vi "V2 Upgrade Refactor Data.vi"() -> (0 "refactor data":T1)   [LabVIEW 2021, in "MeasurementService Editor.lvlib"]
uses:
  MeasurementService Editor.lvlib
  Rename Refactor Mapping Info.ctl
  Rename Refactor Data.ctl
  Rename String Mapping.ctl
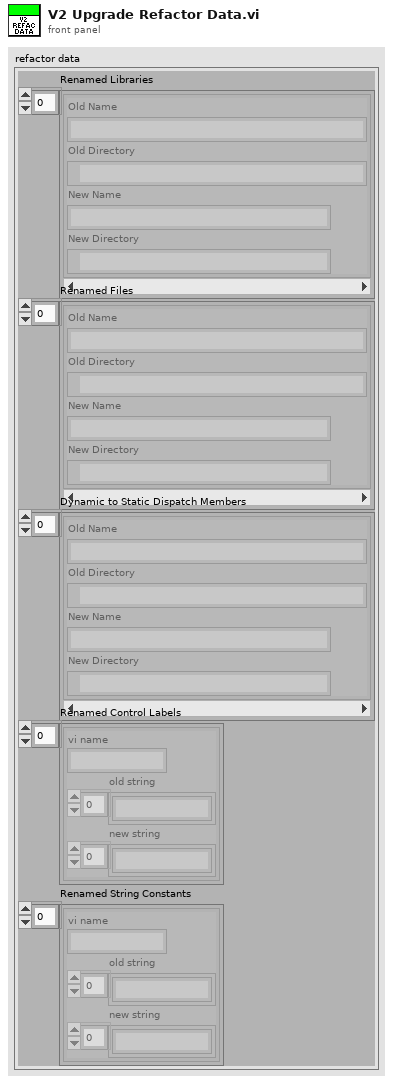
[diagram p1: front panel]
types:
  T1 = typedef "MeasurementService Editor.lvlib/Rename Refactor Data.ctl" = cluster{"Renamed Libraries":T2[], "Renamed Files":T2[], "Dynamic to Static Dispatch Members":T2[], "Renamed Control Labels":T3[], "Renamed String Constants":T3[]}
  T2 = typedef "MeasurementService Editor.lvlib/Rename Refactor Mapping Info.ctl" = cluster{"Old Name":string, "Old Directory":path, "New Name":string, "New Directory":path}
  T3 = typedef "MeasurementService Editor.lvlib/Rename String Mapping.ctl" = cluster{"vi name":string, "old string":string[], "new string":string[]}
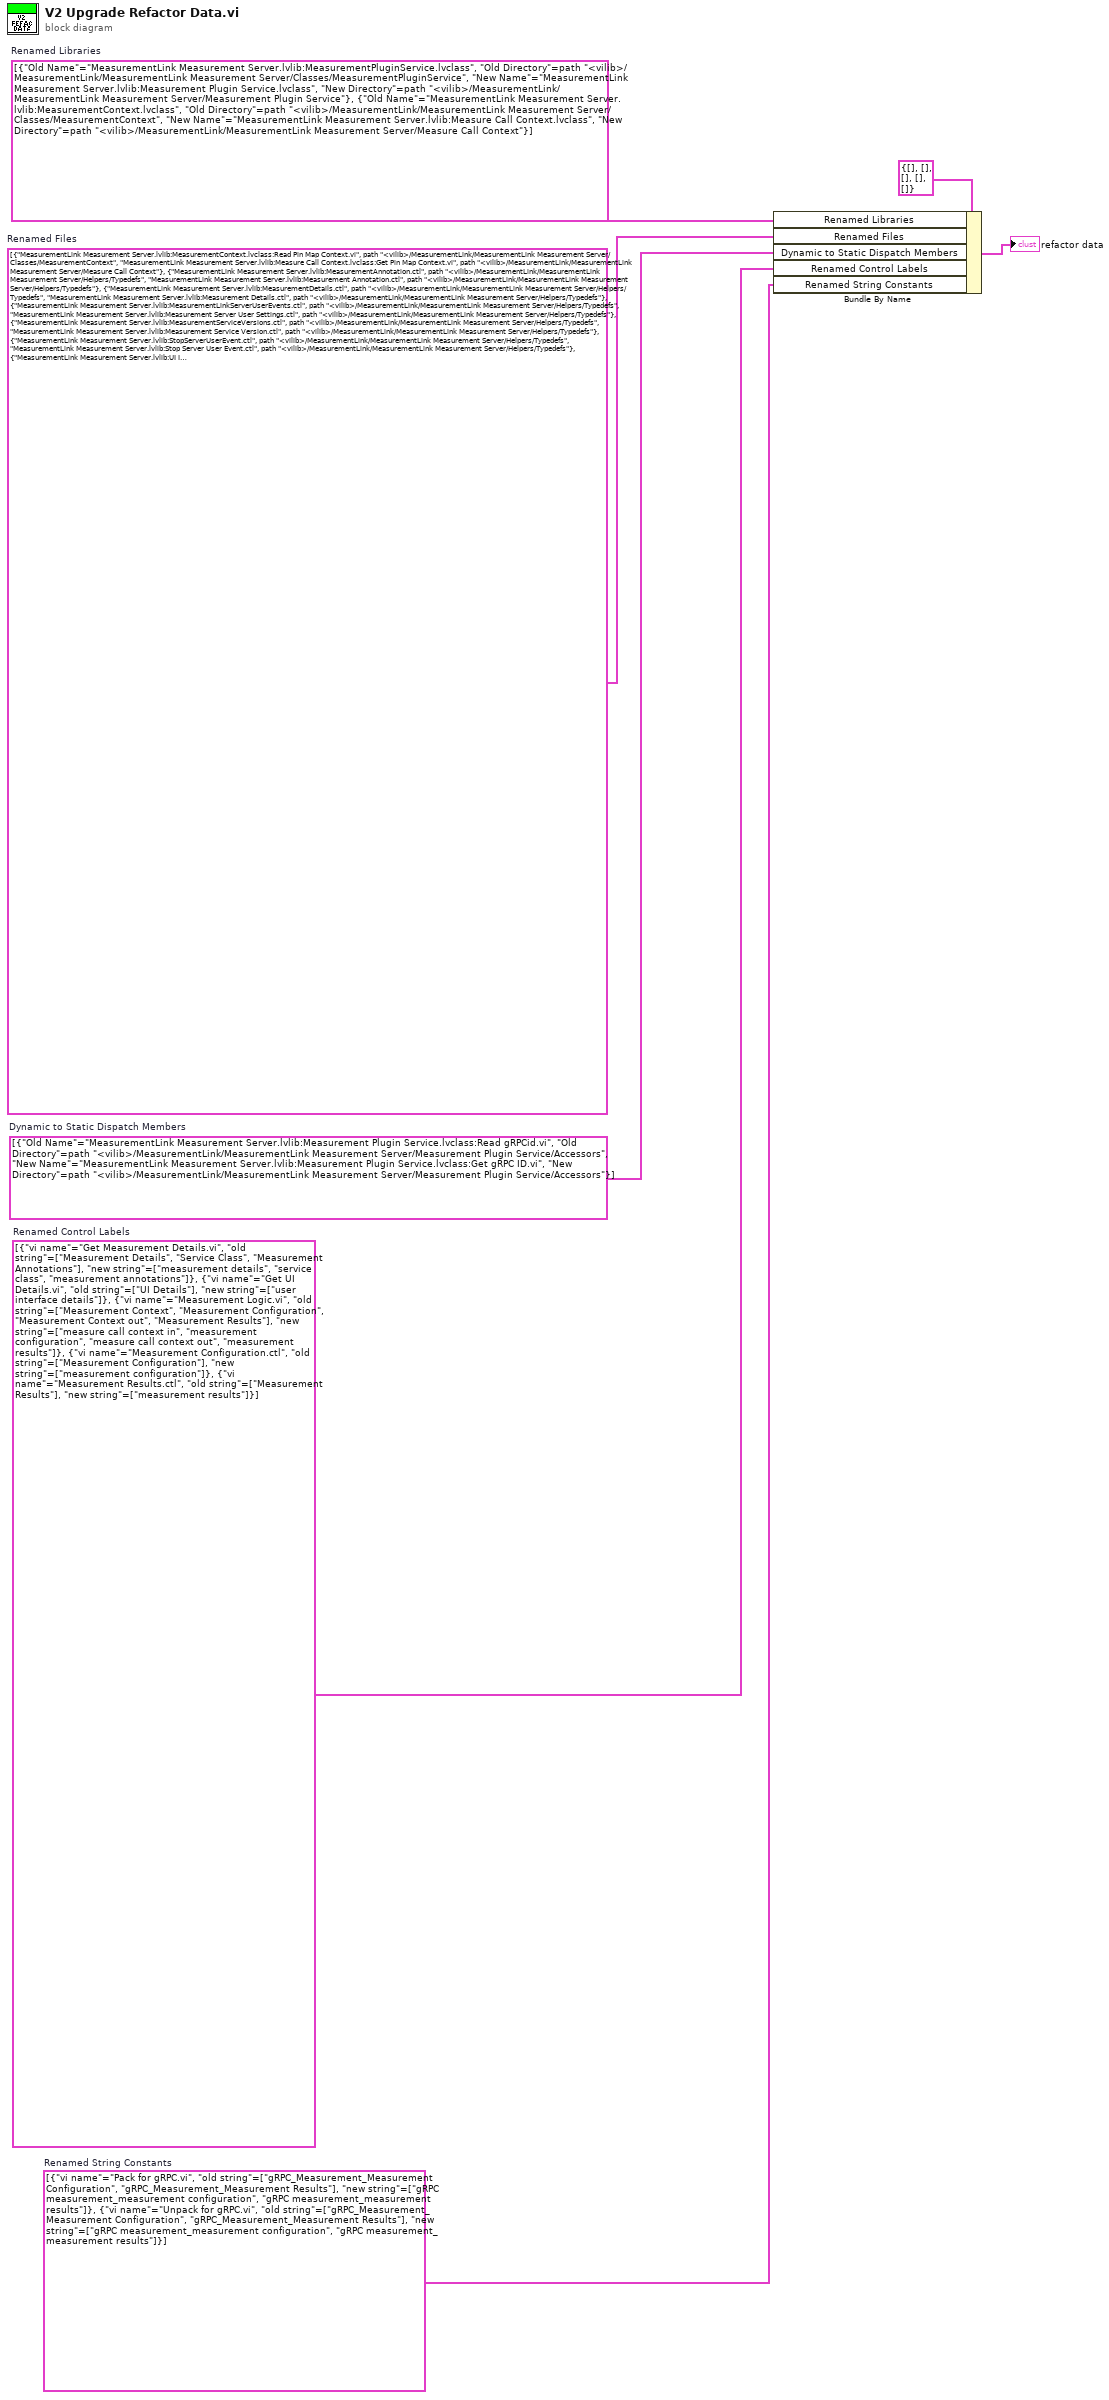
[diagram p0: block diagram]
diagram:
  w1 = T3[] [{"vi name"="Pack for gRPC.vi", "old string"=["gRPC_Measurement_Measurement Configuration", "gRPC_Measurement_Measurement Results"], "new string"=["gRPC measurement_measurement configuration", "gRPC measurement_measurement results"]}, {"vi name"="Unpack for gRPC.vi", "old string"=["gRPC_Measurement_Measurement Configuration", "gRPC_Measurement_Measurement Results"], "new string"=["gRPC measurement_measurement configuration", "gRPC measurement_measurement results"]}]  # Renamed String Constants
  w2 = T3[] [{"vi name"="Get Measurement Details.vi", "old string"=["Measurement Details", "Service Class", "Measurement Annotations"], "new string"=["measurement details", "service class", "measurement annotations"]}, {"vi name"="Get UI Details.vi", "old string"=["UI Details"], "new string"=["user interface details"]}, {"vi name"="Measurement Logic.vi", "old string"=["Measurement Context", "Measurement Configuration", "Measurement Context out", "Measurement Results"], "new string"=["measure call context in", "measurement configuration", "measure call context out", "measurement results"]}, {"vi name"="Measurement Configuration.ctl", "old string"=["Measurement Configuration"], "new string"=["measurement configuration"]}, {"vi name"="Measurement Results.ctl", "old string"=["Measurement Results"], "new string"=["measurement results"]}]  # Renamed Control Labels
  w3 = T2[] [{"Old Name"="MeasurementLink Measurement Server.lvlib:Measurement Plugin Service.lvclass:Read gRPCid.vi", "Old Directory"=path "<vilib>/MeasurementLink/MeasurementLink Measurement Server/Measurement Plugin Service/Accessors", "New Name"="MeasurementLink Measurement Server.lvlib:Measurement Plugin Service.lvclass:Get gRPC ID.vi", "New Directory"=path "<vilib>/MeasurementLink/MeasurementLink Measurement Server/Measurement Plugin Service/Accessors"}]  # Dynamic to Static Dispatch Members
  w4 = T2[] [{"Old Name"="MeasurementLink Measurement Server.lvlib:MeasurementContext.lvclass:Read Pin Map Context.vi", "Old Directory"=path "<vilib>/MeasurementLink/MeasurementLink Measurement Server/Classes/MeasurementContext", "New Name"="MeasurementLink Measurement Server.lvlib:Measure Call Context.lvclass:Get Pin Map Context.vi", "New Directory"=path "<vilib>/MeasurementLink/MeasurementLink Measurement Server/Measure Call Context"}, {"Old Name"="MeasurementLink Measurement Server.lvlib:MeasurementAnnotation.ctl", "Old Directory"=path "<vilib>/MeasurementLink/MeasurementLink Measurement Server/Helpers/Typedefs", "New Name"="MeasurementLink Measurement Server.lvlib:Measurement Annotation.ctl", "New Directory"=path "<vilib>/MeasurementLink/MeasurementLink Measurement Server/Helpers/Typedefs"}, {"Old Name"="MeasurementLink Measurement Server.lvlib:MeasurementDetails.ctl", "Old Directory"=path "<vilib>/MeasurementLink/MeasurementLink Measurement Server/Helpers/Typedefs", "New Name"="MeasurementLink Measurement Server.lvlib:Measurement Details.ctl", "New Directory"=path "<vilib>/MeasurementLink/MeasurementLink Measurement Server/Helpers/Typedefs"}, {"Old Name"="MeasurementLink Measurement Server.lvlib:MeasurementLinkServerUserEvents.ctl", "Old Directory"=path "<vilib>/MeasurementLink/MeasurementLink Measurement Server/Helpers/Typedefs", "New Name"="MeasurementLink Measurement Server.lvlib:Measurement Server User Settings.ctl", "New Directory"=path "<vilib>/MeasurementLink/MeasurementLink Measurement Server/Helpers/Typedefs"}, {"Old Name"="MeasurementLink Measurement Server.lvlib:MeasurementServiceVersions.ctl", "Old Directory"=path "<vilib>/MeasurementLink/MeasurementLink Measurement Server/Helpers/Typedefs", "New Name"="MeasurementLink Measurement Server.lvlib:Measurement Service Version.ctl", "New Directory"=path "<vilib>/MeasurementLink/MeasurementLink Measurement Server/Helpers/Typedefs"}, {"Old Name"="MeasurementLink Measurement Server.lvlib:StopServerUserEvent.ctl", "Old Directory"=path "<vilib>/MeasurementLink/MeasurementLink Measurement Server/Helpers/Typedefs", "New Name"="MeasurementLink Measurement Server.lvlib:Stop Server User Event.ctl", "New Directory"=path "<vilib>/MeasurementLink/MeasurementLink Measurement Server/Helpers/Typedefs"}, {"Old Name"="MeasurementLink Measurement Server.lvlib:UI Information.ctl", "Old Directory"=path "<vilib>/MeasurementLink/MeasurementLink Measurement Server/Helpers/Typedefs", "New Name"="MeasurementLink Measurement Server.lvlib:User Interface Information.ctl", "New Directory"=path "<vilib>/MeasurementLink/MeasurementLink Measurement Server/Helpers/Typedefs"}, {"Old Name"="MeasurementLink Measurement Server.lvlib:Measurement Plugin Service.lvclass:Read gRPCid.vi", "Old Directory"=path "<vilib>/MeasurementLink/MeasurementLink Measurement Server/Measurement Plugin Service/Accessors", "New Name"="MeasurementLink Measurement Server.lvlib:Measurement Plugin Service.lvclass:Get gRPC ID.vi", "New Directory"=path "<vilib>/MeasurementLink/MeasurementLink Measurement Server/Measurement Plugin Service/Accessors"}, {"Old Name"="MeasurementLink Measurement Server.lvlib:Measurement Plugin Service.lvclass:Get UI Details.vi", "Old Directory"=path "<vilib>/MeasurementLink/MeasurementLink Measurement Server/Measurement Plugin Service", "New Name"="MeasurementLink Measurement Server.lvlib:Measurement Plugin Service.lvclass:Get User Interface Details.vi", "New Directory"=path "<vilib>/MeasurementLink/MeasurementLink Measurement Server/Measurement Plugin Service"}, {"Old Name"="MeasurementLink Measurement Server.lvlib:Measurement Plugin Service.lvclass:Pack For Grpc.vi", "Old Directory"=path "<vilib>/MeasurementLink/MeasurementLink Measurement Server/Measurement Plugin Service", "New Name"="MeasurementLink Measurement Server.lvlib:Measurement Plugin Service.lvclass:Pack for gRPC.vi", "New Directory"=path "<vilib>/MeasurementLink/MeasurementLink Measurement Server/Measurement Plugin Service"}, {"Old Name"="MeasurementLink Measurement Server.lvlib:Measurement Plugin Service.lvclass:Unpack For Grpc.vi", "Old Directory"=path "<vilib>/MeasurementLink/MeasurementLink Measurement Server/Measurement Plugin Service", "New Name"="MeasurementLink Measurement Server.lvlib:Measurement Plugin Service.lvclass:Unpack for gRPC.vi", "New Directory"=path "<vilib>/MeasurementLink/MeasurementLink Measurement Server/Measurement Plugin Service"}]  # Renamed Files
  w6 = T2[] [{"Old Name"="MeasurementLink Measurement Server.lvlib:MeasurementPluginService.lvclass", "Old Directory"=path "<vilib>/MeasurementLink/MeasurementLink Measurement Server/Classes/MeasurementPluginService", "New Name"="MeasurementLink Measurement Server.lvlib:Measurement Plugin Service.lvclass", "New Directory"=path "<vilib>/MeasurementLink/MeasurementLink Measurement Server/Measurement Plugin Service"}, {"Old Name"="MeasurementLink Measurement Server.lvlib:MeasurementContext.lvclass", "Old Directory"=path "<vilib>/MeasurementLink/MeasurementLink Measurement Server/Classes/MeasurementContext", "New Name"="MeasurementLink Measurement Server.lvlib:Measure Call Context.lvclass", "New Directory"=path "<vilib>/MeasurementLink/MeasurementLink Measurement Server/Measure Call Context"}]  # Renamed Libraries
  n1 = Bundle By Name(cluster=T1 {"Renamed Libraries"=[], "Renamed Files"=[], "Dynamic to Static Dispatch Members"=[], "Renamed Control Labels"=[], "Renamed String Constants"=[]} ("Rename Data"), "Renamed Libraries"=w6, "Renamed Files"=w4, "Dynamic to Static Dispatch Members"=w3, "Renamed Control Labels"=w2, "Renamed String Constants"=w1) -> (→"refactor data":T1)
